vi "Release Waiting Procs.vi"(8 "error in (no error)":errorcluster, 11 "Notifiers":refnum<queue>[](array[refnum])) -> (0 "Error Out":errorcluster, 3 "Notifiers Out":refnum<queue>[](array[refnum]))   [LabVIEW 2010]
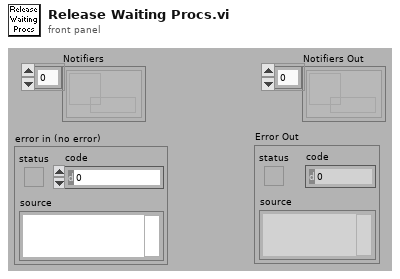
[diagram p1: front panel]
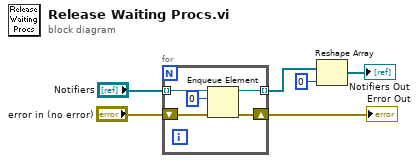
[diagram p0: block diagram]
diagram:
  n1 = for {
    tunnel: "Notifiers" -> [w11] mode=indexing
    shift-right: [w9] -> w6
    shift-left: "error in (no error)" -> [w10]
    tunnel: [w7] -> w3 mode=indexing
    n2 = Enqueue Element(queue=w11, element=0, error in (no error)=w10) -> (queue out=w7:refnum<queue>, error out=w9:errorcluster)  [unwired: 2 out]
  }
  "Error Out" <- w6
  n3 = Reshape Array(w3, 0 ("dimension size")) -> (→"Notifiers Out":refnum<queue>[])
